vi "Loop_ACT_Drive.vi"() -> ()   [LabVIEW 2017]
uses:
  TypeDef/CLUSTER_Drive_HW_SRX_Status.ctl
  TypeDef/CLUSTER_4296_SRX_Status.ctl
  TypeDef/CLUSTER_SRX_Status Data.ctl
  TypeDef/CLUSTER_SRX_Encoder Data.ctl
  TypeDef/CLUSTER_SRX_PWM Data.ctl
  TypeDef/CLUSTER_SRX_Analog Data.ctl
  TypeDef/CLUSTER_SRX_Limit Switch Data.ctl
  TypeDef/CLUSTER_SRX_Profile Data.ctl
  TypeDef/ENUM_Drive_ACT Loop_Mode.ctl
  TypeDef/CLUSTER_Left and Right.ctl
  WCDrive2018/Cluster_WCDrive_SetupData.ctl
  _SHARE ALL/Global Share All/Global_STOP.vi
  Global_SM Write_Data Out.vi
  Global_ACT Write_Data Out.vi
  WCDrive2018/WCDrive2018.lvlib
panel:
  in  "Zero Encoder":bool
  in  "D":dbl
  in  "I":dbl
  in  "P":dbl
  out "Right Data":dbl
  out "Left Data":dbl
  out "Cycle Time (S)":dbl format="%.3g"
  in  "Target Time(ms)":u32=50
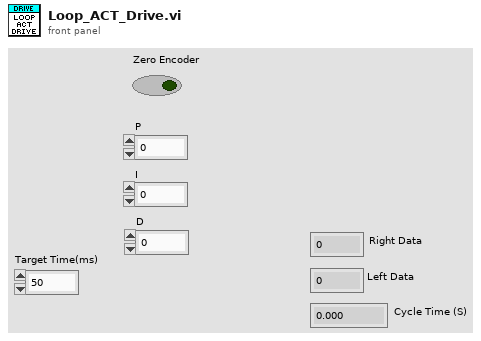
[diagram p1: front panel]
types:
  T1 = typedef "Cluster_WCDrive_SetupData.ctl" = cluster{"Left Master":u8, "Invert Left Master":bool, "Left Slave":u8, "Invert Left Slave":bool, "Right Master":u8, "Invert Right Master":bool, "Right Slave":u8, "Invert Right Slave":bool, "Invert Left Encoder":bool, "Invert Right Encoder":bool}
  T2 = typedef "CLUSTER_Left and Right.ctl" = cluster{"Left":dbl, "Right":dbl}
  T3 = typedef "ENUM_Drive_ACT Loop_Mode.ctl" = enum16{"Stop", "Position", "VBus", "Profile"}
  T4 = typedef "CLUSTER_Drive_HW_SRX_Status.ctl" = cluster{"Rear Left":T5, "Rear Right":T5, "Front Left":T5, "Front Right":T5}
  T5 = typedef "CLUSTER_4296_SRX_Status.ctl" = cluster{"Status":T6, "Encoder":T7, "PWM ":T8, "Analog":T9, "Limit Switches":T10, "Profile":T11}
  T6 = typedef "CLUSTER_SRX_Status Data.ctl" = cluster{"Module Enabled":bool, "Current Profile Slot Select":dbl, "Brake is Enabled":bool, "Applied Throttle":dbl, "Current":dbl, "Battery Voltage":dbl, "Sticky Fault - Under Voltage":bool, "Temperature (C)":dbl, "Sticky Fault - Over Temp":bool, "CAN Error":errorcluster, "Control 5 Is Supported":bool}
  T7 = typedef "CLUSTER_SRX_Encoder Data.ctl" = cluster{"Closed Loop Error":dbl, "Sensor Position":dbl, "Sensor Velocity":dbl, "Encoder Position":dbl, "Encoder Velocity":dbl, "Encoder Index Count":dbl, "Encoder A Pin State":bool, "Encoder B Pin State":bool, "Encoder Index Pin State":bool, "Pos Div 8":bool, "Vel Div 4":bool}
  T8 = typedef "CLUSTER_SRX_PWM Data.ctl" = cluster{"Closed Loop Error":dbl, "Pulse Width Position":i32, "Pulse Width Velocity":i32, "Pulse Width Rise To Rise (us)":i32, "Pulse Width Rise To Fall (us)":i32}
  T9 = typedef "CLUSTER_SRX_Analog Data.ctl" = cluster{"Closed Loop Error":dbl, "Analog In":dbl, "Analog In Velocity":dbl}
  T10 = typedef "CLUSTER_SRX_Limit Switch Data.ctl" = cluster{"Forward Limit Switch Closed":bool, "Reverse Limit Switch Closed":bool, "Sticky Fault - Forward Limit":bool, "Sticky Fault - Reverse Limit":bool, "Sticky Fault - Forward Soft Limit":bool, "Sticky Fault - Reverse Soft Limit":bool}
  T11 = typedef "CLUSTER_SRX_Profile Data.ctl" = cluster{"Mot Prof Active Is Under Run":bool, "Mot Prof Active Has Under Run":bool, "Mot Prof Active Is Last":bool, "Mot Prof Active Velocity Only":bool, "Mot Prof Active Is Valid":bool, "Mot Prof Buffer Is Full":bool, "Mot Prof Active Profile Slot Select":i32, "Mot Prof NextID":i32, "Mot Prof Count":i32, "Mot Prof Active Velocity":dbl, "Mot Prof Active Position":dbl, "Mot Prof Output Enable":i32}
  T12 = typedef "WPI_RobotDriveDevRef.ctl" = cluster{"DevStatus":errorcluster, "Motors[]":T13[], "Square Inputs":bool, "Max Output":dbl}
  T13 = typedef "WPI_MotorControlDeviceRef.ctl" = cluster{"DeviceStatus":errorcluster, "Type":T14, "PWM":cluster{"PWM Channel":T15, "DeadBand":T16}, "CAN":cluster{"Device Number":u8, "SetOutput VI Ref":variant, "GetOutput VI Ref":variant, "Enable VI Ref":variant, "Disable VI Ref":variant, "Data":variant}, "Invert":bool, "DIO PWM":cluster{"PWM \"Enable\" Channel":T15, "DIOChannel":T17, "PWM Rate":dbl}}
  T14 = typedef "WPI_MotorControlType.ctl" = enum16{"PWM", "CAN", "DIO PWM"}
  T15 = typedef "FPGA_DIOPWMChannel.ctl" = enum8{"PWM 0", "PWM 1", "PWM 2", "PWM 3", "PWM 4", "PWM 5", "PWM 6", "PWM 7", "PWM 8", "PWM 9", "PWM MXP 0", "PWM MXP 1", "PWM MXP 2", "PWM MXP 3", "PWM MXP 4", "PWM MXP 5", "PWM MXP 6", "PWM MXP 7", "PWM MXP 8", "PWM MXP 9", "Invalid"}
  T16 = typedef "WPI_PWMDeadband.ctl" = cluster{"Name":string, "maxPositivePwm":i32, "minPositivePwm":i32, "centerPwm":i32, "maxNegativePwm":i32, "minNegativePwm":i32, "angularRange":u16}
  T17 = typedef "FPGA_DIOChannel.ctl" = enum8{"DIO 0", "DIO 1", "DIO 2", "DIO 3", "DIO 4", "DIO 5", "DIO 6", "DIO 7", "DIO 8", "DIO 9", "DIO MXP 0", "DIO MXP 1", "DIO MXP 2", "DIO MXP 3", "DIO MXP 4", "DIO MXP 5", "DIO MXP 6", "DIO MXP 7", "DIO MXP 8", "DIO MXP 9", "DIO MXP 10", "DIO MXP 11", "DIO MXP 12", "DIO MXP 13", "DIO MXP 14", "DIO MXP 15", "SPI Port CS1", "SPI Port CS2", "SPI Port CS3", "SPI Port MISO", "SPI Port MOSI", "Invalid"}
  T18 = cluster{"RobotDriveDevRef Out":T12, "Target Time(ms)":u32, "Current Time":timestamp, "Previous Time":timestamp, "Cycle Time (S)":dbl, "SRX_Status":T4, "Mode":T3, "VBus":T2, "Cruise RPM":dbl, "MAX Velocity\n":dbl, "Encoder Target Position":i32, "Zero Encoder":bool}
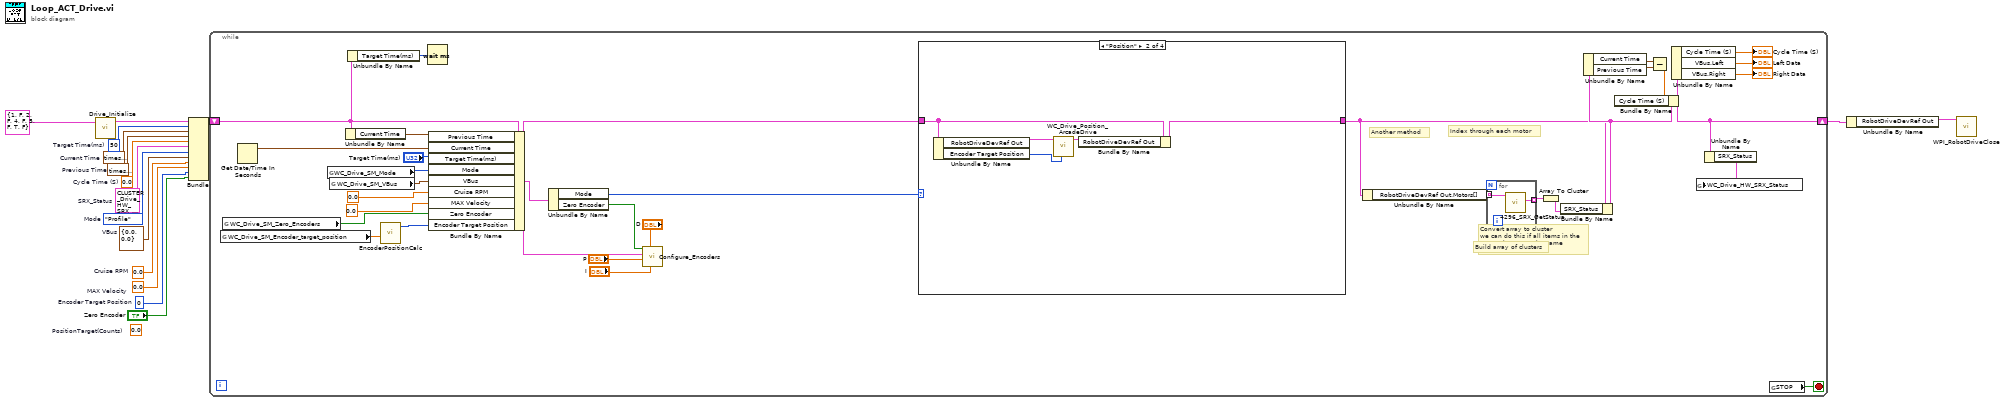
[diagram p0: block diagram]
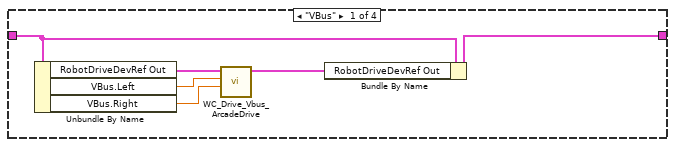
[diagram p2: hidden frame]
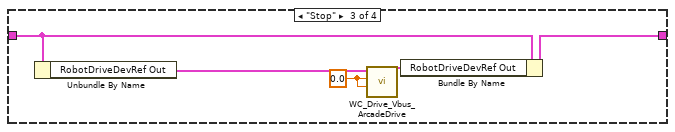
[diagram p3: hidden frame]
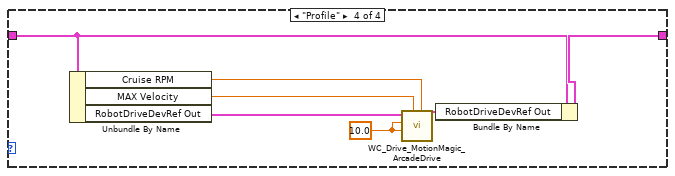
[diagram p4: hidden frame]
diagram:
  (unwired) 0.0  # PositionTarget(Counts)
  w4 = 0  # Encoder Target Position
  w5 = 0.0  # MAX Velocity
  w6 = 0.0  # Cruise RPM
  w7 = T2 {"Left"=0.0, "Right"=0.0}  # VBus
  w8 = ENUM_Drive_ACT_Loop_Mode."Profile"  # Mode
  w9 = T4 {"Rear Left"={"Status"={"Module Enabled"=FALSE, "Current Profile Slot Select"=0.0, "Brake is Enabled"=FALSE, "Applied Throttle"=0.0, "Current"=0.0, "Battery Voltage"=0.0, "Sticky Fault - Under Voltage"=FALSE, "Temperature (C)"=0.0, "Sticky Fault - Over Temp"=FALSE, "CAN Error"={"status"=FALSE, "code"=0, "source"=""}, "Control 5 Is Supported"=FALSE}, "Encoder"={"Closed Loop Error"=0.0, "Sensor Position"=0.0, "Sensor Velocity"=0.0, "Encoder Position"=0.0, "Encoder Velocity"=0.0, "Encoder Index Count"=0.0, "Encoder A Pin State"=FALSE, "Encoder B Pin State"=FALSE, "Encoder Index Pin State"=FALSE, "Pos Div 8"=FALSE, "Vel Div 4"=FALSE}, "PWM "={"Closed Loop Error"=0.0, "Pulse Width Position"=0, "Pulse Width Velocity"=0, "Pulse Width Rise To Rise (us)"=0, "Pulse Width Rise To Fall (us)"=0}, "Analog"={"Closed Loop Error"=0.0, "Analog In"=0.0, "Analog In Velocity"=0.0}, "Limit Switches"={"Forward Limit Switch Closed"=FALSE, "Reverse Limit Switch Closed"=FALSE, "Sticky Fault - Forward Limit"=FALSE, "Sticky Fault - Reverse Limit"=FALSE, "Sticky Fault - Forward Soft Limit"=FALSE, "Sticky Fault - Reverse Soft Limit"=FALSE}, "Profile"={"Mot Prof Active Is Under Run"=FALSE, "Mot Prof Active Has Under Run"=FALSE, "Mot Prof Active Is Last"=FALSE, "Mot Prof Active Velocity Only"=FALSE, "Mot Prof Active Is Valid"=FALSE, "Mot Prof Buffer Is Full"=FALSE, "Mot Prof Active Profile Slot Select"=0, "Mot Prof NextID"=0, "Mot Prof Count"=0, "Mot Prof Active Velocity"=0.0, "Mot Prof Active Position"=0.0, "Mot Prof Output Enable"=0}}, "Rear Right"={"Status"={"Module Enabled"=FALSE, "Current Profile Slot Select"=0.0, "Brake is Enabled"=FALSE, "Applied Throttle"=0.0, "Current"=0.0, "Battery Voltage"=0.0, "Sticky Fault - Under Voltage"=FALSE, "Temperature (C)"=0.0, "Sticky Fault - Over Temp"=FALSE, "CAN Error"={"status"=FALSE, "code"=0, "source"=""}, "Control 5 Is Supported"=FALSE}, "Encoder"={"Closed Loop Error"=0.0, "Sensor Position"=0.0, "Sensor Velocity"=0.0, "Encoder Position"=0.0, "Encoder Velocity"=0.0, "Encoder Index Count"=0.0, "Encoder A Pin State"=FALSE, "Encoder B Pin State"=FALSE, "Encoder Index Pin State"=FALSE, "Pos Div 8"=FALSE, "Vel Div 4"=FALSE}, "PWM "={"Closed Loop Error"=0.0, "Pulse Width Position"=0, "Pulse Width Velocity"=0, "Pulse Width Rise To Rise (us)"=0, "Pulse Width Rise To Fall (us)"=0}, "Analog"={"Closed Loop Error"=0.0, "Analog In"=0.0, "Analog In Velocity"=0.0}, "Limit Switches"={"Forward Limit Switch Closed"=FALSE, "Reverse Limit Switch Closed"=FALSE, "Sticky Fault - Forward Limit"=FALSE, "Sticky Fault - Reverse Limit"=FALSE, "Sticky Fault - Forward Soft Limit"=FALSE, "Sticky Fault - Reverse Soft Limit"=FALSE}, "Profile"={"Mot Prof Active Is Under Run"=FALSE, "Mot Prof Active Has Under Run"=FALSE, "Mot Prof Active Is Last"=FALSE, "Mot Prof Active Velocity Only"=FALSE, "Mot Prof Active Is Valid"=FALSE, "Mot Prof Buffer Is Full"=FALSE, "Mot Prof Active Profile Slot Select"=0, "Mot Prof NextID"=0, "Mot Prof Count"=0, "Mot Prof Active Velocity"=0.0, "Mot Prof Active Position"=0.0, "Mot Prof Output Enable"=0}}, "Front Left"={"Status"={"Module Enabled"=FALSE, "Current Profile Slot Select"=0.0, "Brake is Enabled"=FALSE, "Applied Throttle"=0.0, "Current"=0.0, "Battery Voltage"=0.0, "Sticky Fault - Under Voltage"=FALSE, "Temperature (C)"=0.0, "Sticky Fault - Over Temp"=FALSE, "CAN Error"={"status"=FALSE, "code"=0, "source"=""}, "Control 5 Is Supported"=FALSE}, "Encoder"={"Closed Loop Error"=0.0, "Sensor Position"=0.0, "Sensor Velocity"=0.0, "Encoder Position"=0.0, "Encoder Velocity"=0.0, "Encoder Index Count"=0.0, "Encoder A Pin State"=FALSE, "Encoder B Pin State"=FALSE, "Encoder Index Pin State"=FALSE, "Pos Div 8"=FALSE, "Vel Div 4"=FALSE}, "PWM "={"Closed Loop Error"=0.0, "Pulse Width Position"=0, "Pulse Width Velocity"=0, "Pulse Width Rise To Rise (us)"=0, "Pulse Width Rise To Fall (us)"=0}, "Analog"={"Closed Loop Error"=0.0, "Analog In"=0.0, "Analog In Velocity"=0.0}, "Limit Switches"={"Forward Limit Switch Closed"=FALSE, "Reverse Limit Switch Closed"=FALSE, "Sticky Fault - Forward Limit"=FALSE, "Sticky Fault - Reverse Limit"=FALSE, "Sticky Fault - Forward Soft Limit"=FALSE, "Sticky Fault - Reverse Soft Limit"=FALSE}, "Profile"={"Mot Prof Active Is Under Run"=FALSE, "Mot Prof Active Has Under Run"=FALSE, "Mot Prof Active Is Last"=FALSE, "Mot Prof Active Velocity Only"=FALSE, "Mot Prof Active Is Valid"=FALSE, "Mot Prof Buffer Is Full"=FALSE, "Mot Prof Active Profile Slot Select"=0, "Mot Prof NextID"=0, "Mot Prof Count"=0, "Mot Prof Active Velocity"=0.0, "Mot Prof Active Position"=0.0, "Mot Prof Output Enable"=0}}, "Front Right"={"Status"={"Module Enabled"=FALSE, "Current Profile Slot Select"=0.0, "Brake is Enabled"=FALSE, "Applied Throttle"=0.0, "Current"=0.0, "Battery Voltage"=0.0, "Sticky Fault - Under Voltage"=FALSE, "Temperature (C)"=0.0, "Sticky Fault - Over Temp"=FALSE, "CAN Error"={"status"=FALSE, "code"=0, "source"=""}, "Control 5 Is Supported"=FALSE}, "Encoder"={"Closed Loop Error"=0.0, "Sensor Position"=0.0, "Sensor Velocity"=0.0, "Encoder Position"=0.0, "Encoder Velocity"=0.0, "Encoder Index Count"=0.0, "Encoder A Pin State"=FALSE, "Encoder B Pin State"=FALSE, "Encoder Index Pin State"=FALSE, "Pos Div 8"=FALSE, "Vel Div 4"=FALSE}, "PWM "={"Closed Loop Error"=0.0, "Pulse Width Position"=0, "Pulse Width Velocity"=0, "Pulse Width Rise To Rise (us)"=0, "Pulse Width Rise To Fall (us)"=0}, "Analog"={"Closed Loop Error"=0.0, "Analog In"=0.0, "Analog In Velocity"=0.0}, "Limit Switches"={"Forward Limit Switch Closed"=FALSE, "Reverse Limit Switch Closed"=FALSE, "Sticky Fault - Forward Limit"=FALSE, "Sticky Fault - Reverse Limit"=FALSE, "Sticky Fault - Forward Soft Limit"=FALSE, "Sticky Fault - Reverse Soft Limit"=FALSE}, "Profile"={"Mot Prof Active Is Under Run"=FALSE, "Mot Prof Active Has Under Run"=FALSE, "Mot Prof Active Is Last"=FALSE, "Mot Prof Active Velocity Only"=FALSE, "Mot Prof Active Is Valid"=FALSE, "Mot Prof Buffer Is Full"=FALSE, "Mot Prof Active Profile Slot Select"=0, "Mot Prof NextID"=0, "Mot Prof Count"=0, "Mot Prof Active Velocity"=0.0, "Mot Prof Active Position"=0.0, "Mot Prof Output Enable"=0}}}  # SRX_Status
  w11 = 0.0  # Cycle Time (S)
  w16 = timestamp(0 s since 1904-01-01)  # Previous Time
  w15 = timestamp(0 s since 1904-01-01)  # Current Time
  w14 = u32 50  # Target Time(ms)
  n1 = call "Drive_Initialize.vi"("HW SETUP_WC Drive"=T1 {"Left Master"=1, "Invert Left Master"=FALSE, "Left Slave"=2, "Invert Left Slave"=FALSE, "Right Master"=4, "Invert Right Master"=FALSE, "Right Slave"=5, "Invert Right Slave"=FALSE, "Invert Left Encoder"=TRUE, "Invert Right Encoder"=FALSE}) -> ("RobotDriveDevRef Out"=w3:T12)  [unwired: 10 in]
  n2 = Bundle("RobotDriveDevRef Out"=w3, "Target Time(ms)"=w14, "Current Time"=w15, "Previous Time"=w16, "Cycle Time (S)"=w11, "SRX_Status"=w9, "Mode"=w8, "VBus"=w7, "Cruise RPM"=w6, "MAX Velocity"=w5, "Encoder Target Position"=w4, "Zero Encoder"="Zero Encoder") -> (w13:T18)  [unwired: 1 in]
  n3 = while {
    shift-right: [w34] -> w12
    shift-left: w13 -> [w31]
    stop <- w48 stop-if-true
    # "Build array of clusters"
    # "Convert array to cluster\nwe can do this if all items in the\nstatus cluster are the same"
    # "Index through each motor"
    # "Another method"
    n4 = global read "Global_SM Write_Data Out.vi" "WC_Drive_SM_Encoder_target_position"() -> (w20:dbl)
    n5 = global read "Global_SM Write_Data Out.vi" "WC_Drive_SM_Zero_Encoders"() -> (w22:bool)
    n6 = Get Date/Time In Seconds() -> (seconds since 1Jan1904=w47:timestamp)
    n7 = global read "Global_SM Write_Data Out.vi" "WC_Drive_SM_Mode"() -> (w37:T3)
    n8 = global read "Global_SM Write_Data Out.vi" "WC_Drive_SM_VBus"() -> (w30:T2)
    n9 = Unbundle By Name(w31) -> ("Current Time"=w46:timestamp)
    n10 = Unbundle By Name(w31) -> ("Target Time(ms)"=w42:u32)
    n11 = call "EncoderPositionCalc.vi"("PositionTarget(in)"=w20) -> ("PostionTarget(Counts)"=w21:i32)  [unwired: 10 in]
    n12 = Wait (ms)(milliseconds to wait=w42) -> ()  [unwired: 1 out]
    n13 = Bundle By Name(cluster=w31, "Previous Time"=w46, "Current Time"=w47, "Target Time(ms)"="Target Time(ms)", "Mode"=w37, "VBus"=w30, "Cruise RPM"=0.0, "MAX Velocity"=0.0, "Zero Encoder"=w22, "Encoder Target Position"=w21) -> (w27:T18)
    n14 = Unbundle By Name(w27) -> ("Mode"=w36:T3, "Zero Encoder"=w23:bool)
    n15 = call "Configure_Encoders.vi"("I"="I", "D"="D", "P"="P", "Cluster"=w27, "Zero Encoder"=w23) -> ()  [unwired: 7 in]
    n16 = case shown="\"Position\"" w36 {
      tunnel: w27 -> [w52 w61 w65 w69]
      tunnel: [w51 w60 w64 w70] -> w32
      frame "VBus" {
        n17 = Unbundle By Name(w52) -> ("RobotDriveDevRef Out"=w56:T12, "VBus.Left"=w55:dbl, "VBus.Right"=w54:dbl)
        n18 = call "WC_Drive_Vbus_ArcadeDrive.vi"("Right Value"=w54, "Left Value"=w55, "RobotDriveDevRef"=w56) -> ("RobotDriveDevRef Out"=w53:T12)  [unwired: 7 in, 1 out]
        n19 = Bundle By Name(cluster=w52, "RobotDriveDevRef Out"=w53) -> (w51:T18)
      }
      frame "Position" {
        n20 = Unbundle By Name(w61) -> ("RobotDriveDevRef Out"=w59:T12, "Encoder Target Position"=w57:i32)
        n21 = call "WC_Drive_Position_ArcadeDrive.vi"("Encoder Target Position"=w57, "RobotDriveDevRef"=w59) -> ("RobotDriveDevRef Out"=w58:T12)  [unwired: 8 in, 1 out]
        n22 = Bundle By Name(cluster=w61, "RobotDriveDevRef Out"=w58) -> (w60:T18)
      }
      frame "Stop" {
        w63 = 0.0 ("X axis value")
        n23 = Unbundle By Name(w65) -> ("RobotDriveDevRef Out"=w62:T12)
        n24 = call "WC_Drive_Vbus_ArcadeDrive.vi"("Right Value"=w63, "Left Value"=w63, "RobotDriveDevRef"=w62) -> ("RobotDriveDevRef Out"=w66:T12)  [unwired: 7 in, 1 out]
        n25 = Bundle By Name(cluster=w65, "RobotDriveDevRef Out"=w66) -> (w64:T18)
      }
      frame "Profile" {
        w72 = 10.0 ("X axis value")
        n26 = Unbundle By Name(w69) -> ("Cruise RPM"=w68:dbl, "MAX Velocity"=w67:dbl, "RobotDriveDevRef Out"=w73:T12)
        n27 = call "WC_Drive_MotionMagic_ArcadeDrive.vi"("Cruise RPM"=w68, "Max Velocity"=w67, "Right Value"=w72, "Left Value"=w72, "RobotDriveDevRef"=w73) -> ("RobotDriveDevRef Out"=w71:T12)  [unwired: 5 in, 1 out]
        n28 = Bundle By Name(cluster=w69, "RobotDriveDevRef Out"=w71) -> (w70:T18)
      }
    }
    n29 = Unbundle By Name(w32) -> ("RobotDriveDevRef Out.Motors[]"=w19:T13[])
    n30 = for {
      tunnel: w19 -> [w50] mode=indexing
      tunnel: [w49] -> w18 mode=indexing
      n31 = call "4296_SRX_GetStatus.vi"("CAN Talon SRX Ref"=w50) -> ("4296 SRX Status Out"=w49:T5)  [unwired: 8 in, 2 out]
    }
    n32 = Array To Cluster(array=w18) -> (cluster=w17:cluster{"[0]":T5, "[1]":T5, "[2]":T5, "[3]":T5})
    n33 = Bundle By Name(cluster=w32, "SRX_Status"=w17) -> (w33:T18)
    n34 = Unbundle By Name(w33) -> ("Current Time"=w45:timestamp, "Previous Time"=w44:timestamp)
    n35 = Subtract(x=w45, y=w44) -> (x-y=w35:dbl)
    n36 = Bundle By Name(cluster=w33, "Cycle Time (S)"=w35) -> (w34:T18)
    n37 = Unbundle By Name(w34) -> ("Cycle Time (S)"=→"Cycle Time (S)":dbl, "VBus.Left"=→"Left Data":dbl, "VBus.Right"=→"Right Data":dbl)
    n38 = Unbundle By Name(w34) -> ("SRX_Status"=w38:T4)
    n39 = global write "Global_ACT Write_Data Out.vi" "WC_Drive_HW_SRX_Status"(w38) -> ()
    n40 = global read "Global_STOP.vi" "STOP"() -> (w48:bool)
  }
  n41 = Unbundle By Name(w12) -> ("RobotDriveDevRef Out"=w10:T12)
  n42 = call <vilib>:"WPI_RobotDriveClose.vi"("RobotDriveDevRef"=w10) -> ()  [unwired: 10 in, 1 out]
